vi "Command Type.vi"(11 "Digital Command Config in":refnum<class "Digital Command Config.lvclass">) -> (2 "Command Type":string)   [LabVIEW 2020, in "VolatusSeqConfig.lvlib" / "Digital Command Config.lvclass"]
uses:
  Digital Command Config.lvclass
  Digital Command Config.lvclass/Digital Command Config.ctl
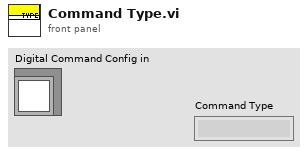
[diagram p1: front panel]
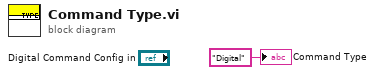
[diagram p0: block diagram]
diagram:
  "Command Type" <- "Digital" ("Command Type")
